vi "U6 Single AIN Example.vi"() -> (0 "error out":errorcluster)   [LabVIEW 2021]
panel:
  in  "Negative Channel #":i32=199
  in  "AIN Range":u16(ring) items=["LJ_rgBIP10V", "LJ_rgBIP1V", "LJ_rgBIPP1V", "LJ_rgBIPP01V"]
  in  "Binary":bool
  in  "SettlingFactor":i32
  in  "Resolution":i32
  in  "FirstFound":bool=TRUE
  in  "Address":string="1"
  out "Error Message":string
  out "Value Read":dbl format="%.9f"
  in  "Positive Channel #":i32
  # "Configures and reads 1 analog input."
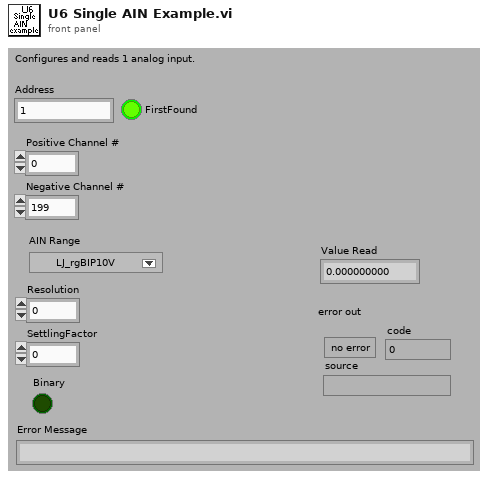
[diagram p1: front panel]
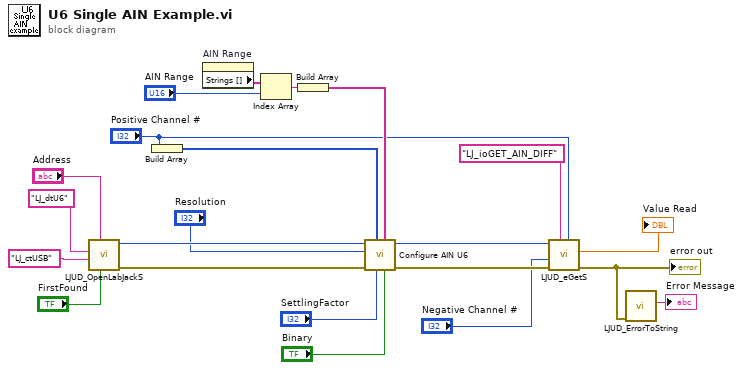
[diagram p0: block diagram]
diagram:
  n1 = call "LJUD_OpenLabJackS.vi"("FirstFound"="FirstFound", "Address"="Address", "ConnectionType"="LJ_ctUSB", "DeviceType"="LJ_dtU6") -> ("error out"=w11:errorcluster, "Handle"=w12:i32)  [unwired: 5 in, 1 out]
  n2 = Build Array("Positive Channel #") -> (w8:i32[])
  n3 = property on="AIN Range" class="Ring (strict)"() -> ("Strings []"=w10:string[])  [unwired: 2 in, 2 out]
  n4 = Index Array(array=w10, index="AIN Range") -> (element=w7:string)
  n5 = Build Array(w7) -> (w6:string[])
  n6 = call "Configure AIN U6.vi"("Binary"="Binary", "Ranges"=w6, "SettlingFactor"="SettlingFactor", "Positive Channels"=w8, "error in"=w11, "Resolution"="Resolution", "Handle In"=w12) -> ("error out"=w14:errorcluster, "Handle Out"=w13:i32)  [unwired: 3 in]
  n7 = call "LJUD_eGetS.vi"("Channel"="Positive Channel #", "IOType"="LJ_ioGET_AIN_DIFF", "error in"=w14, "x1"="Negative Channel #", "Handle In"=w13) -> ("error out"=w19:errorcluster, "Value Read"=→"Value Read":dbl)  [unwired: 4 in, 1 out]
  "error out" <- w19
  n8 = call "LJUD_ErrorToString.vi"("error in"=w19) -> ("String"=→"Error Message":string)  [unwired: 10 in]
